vi "ExampleClient.vi"() -> ()   [LabVIEW 2017]
uses:
  Support/StreamClientState.ctl
  Controller/Support/StreamHeader.ctl
  jsonRPCwebservice/client/config.ctl
  Support/msg.ctl
  <userlib>/_SEH/Controls/CEH/CEH Actions.ctl
  <vilib>/NI/JSON Support for LabVIEW/JSON Data Classes/JSON String/JSON String.lvclass
  C:/Program Files (x86)/National Instruments/LabVIEW 2017/vi.lib/NI/JSON Support for LabVIEW/JSON Data Classes/JSON Datatype/JSON Null.lvclass
  Support/client_globals.vi
  jsonRPCwebservice/client/Request_int_JSON.vi
  <vilib>/NI/JSON Support for LabVIEW/JSON Data Classes/JSON Helper/To More Specific Type (Object).vi
  <vilib>/NI/JSON Support for LabVIEW/JSON Data Classes/JSON Object/Get Value (String).vi
  <vilib>/NI/JSON Support for LabVIEW/JSON Data Classes/JSON String/Read value (String).vi
  <vilib>/NI/JSON Support for LabVIEW/JSON Data Classes/JSON String/New JSON String.vi
  <vilib>/NI/JSON Support for LabVIEW/JSON Data Classes/JSON Helper/Parsing/Parse Value.vi
  <vilib>/NI/JSON Support for LabVIEW/JSON Data Classes/JSON Object/Get Value (Array).vi
  <vilib>/NI/JSON Support for LabVIEW/JSON Data Classes/JSON Array/Index Array XNode/index helper.vi
  <vilib>/NI/JSON Support for LabVIEW/JSON Data Classes/JSON Array/Index Array.vi
  <vilib>/NI/JSON Support for LabVIEW/JSON Data Classes/JSON Array/Index Array (JSON).vi
  <vilib>/NI/JSON Support for LabVIEW/JSON Data Classes/JSON Helper/To More Specific Type (Array).vi
  <vilib>/NI/JSON Support for LabVIEW/JSON Data Classes/JSON Array/Get Array Values as Strings.vi
  <vilib>/WebDAVClient/Simple Get File.vi
  <vilib>/NI/JSON Support for LabVIEW/JSON Data Classes/JSON Datatype/JSON Null.lvclass
  <vilib>/NI/JSON Support for LabVIEW/JSON Data Classes/JSON Array/Index Array XNode/Index JSON Array.xnode
  <vilib>/NI/JSON Support for LabVIEW/JSON Data Classes/JSON Array/JSON Array.lvclass
  jsonRPCwebservice/client/JSON_RPC_client.lvlib
  <vilib>/WebDAVClient/NI_WebDAV.lvlib
  <vilib>/NI/JSON Support for LabVIEW/JSON Data Classes/JSON Helper/JSON Helper.lvclass
  <vilib>/NI/JSON Support for LabVIEW/JSON Data Classes/JSON Object/JSON Object.lvclass
  <vilib>/NI/JSON Support for LabVIEW/JSON Data Classes/JSON Basic Type/JSON Literal.lvclass
panel:
  in  "Trace":string
  in  "Tab Control":enum32{"Commands", "Stream", "Files"}(tab)
  in  "ClearSafeState":bool
  in  "ToEcho":string
  in  "CheckConnection":bool
  in  "GoToSafeState":bool
  in  "GetResourceUsage":bool
  in  "echo":bool
  out "Current State":string
  out "logging":bool
  out "Waveforms":sgl[][](graph)
  in  "Stream":bool
  in  "StreamAndLog":bool
  in  "StopStreaming":bool
  in  "ForceTigger":bool
  in  "RefreshLogFiles":bool
  in  "Logs":i32(listbox)
  in  "Download":bool
  in  "Exit":bool
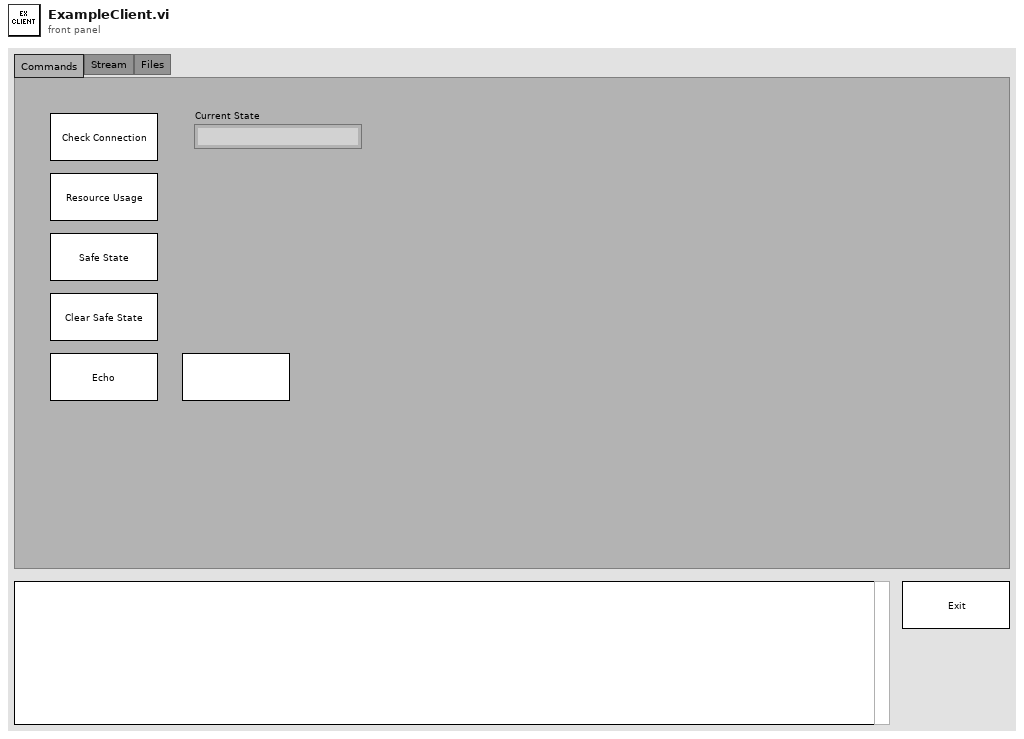
[diagram p1: front panel]
types:
  T1 = typedef "msg.ctl" = cluster{"cmd":string, "parameters":variant}
  T2 = typedef "JSON_RPC_client.lvlib/config.ctl" = cluster{"ip":string, "port":i32, "username":string, "password":string}
  T3 = typedef "StreamHeader.ctl" = cluster{"Channels":string[], "SampleRate":i32}
  T4 = typedef "StreamClientState.ctl" = enum16{"Initialize", "Idle", "ConnectAndOpen", "Connecting", "ReadHeader", "Streaming", "Disconnecting"}
  T5 = enum8{"Enabled", "Disabled", "Disabled and Grayed Out"}
  T6 = typedef "JSON_RPC_client.lvlib/reference.ctl" = cluster{"client handle":T7, "url":string}
  T7 = typedef "LabVIEWHTTPClient.lvlib/ClientHandle.ctl" = refnum<k1>
  T8 = enum16{"open", "open or create", "create or replace", "create", "open (read-only)"}
  T9 = typedef "SEH Notification Info.ctl" = cluster{"Priority":i32, "Occurrences":i32, "First Occurrence":timestamp}
  T10 = typedef "CEH Actions.ctl" = enum16{"Log", "Display Error Message", "Safe State", "Shutdown"}
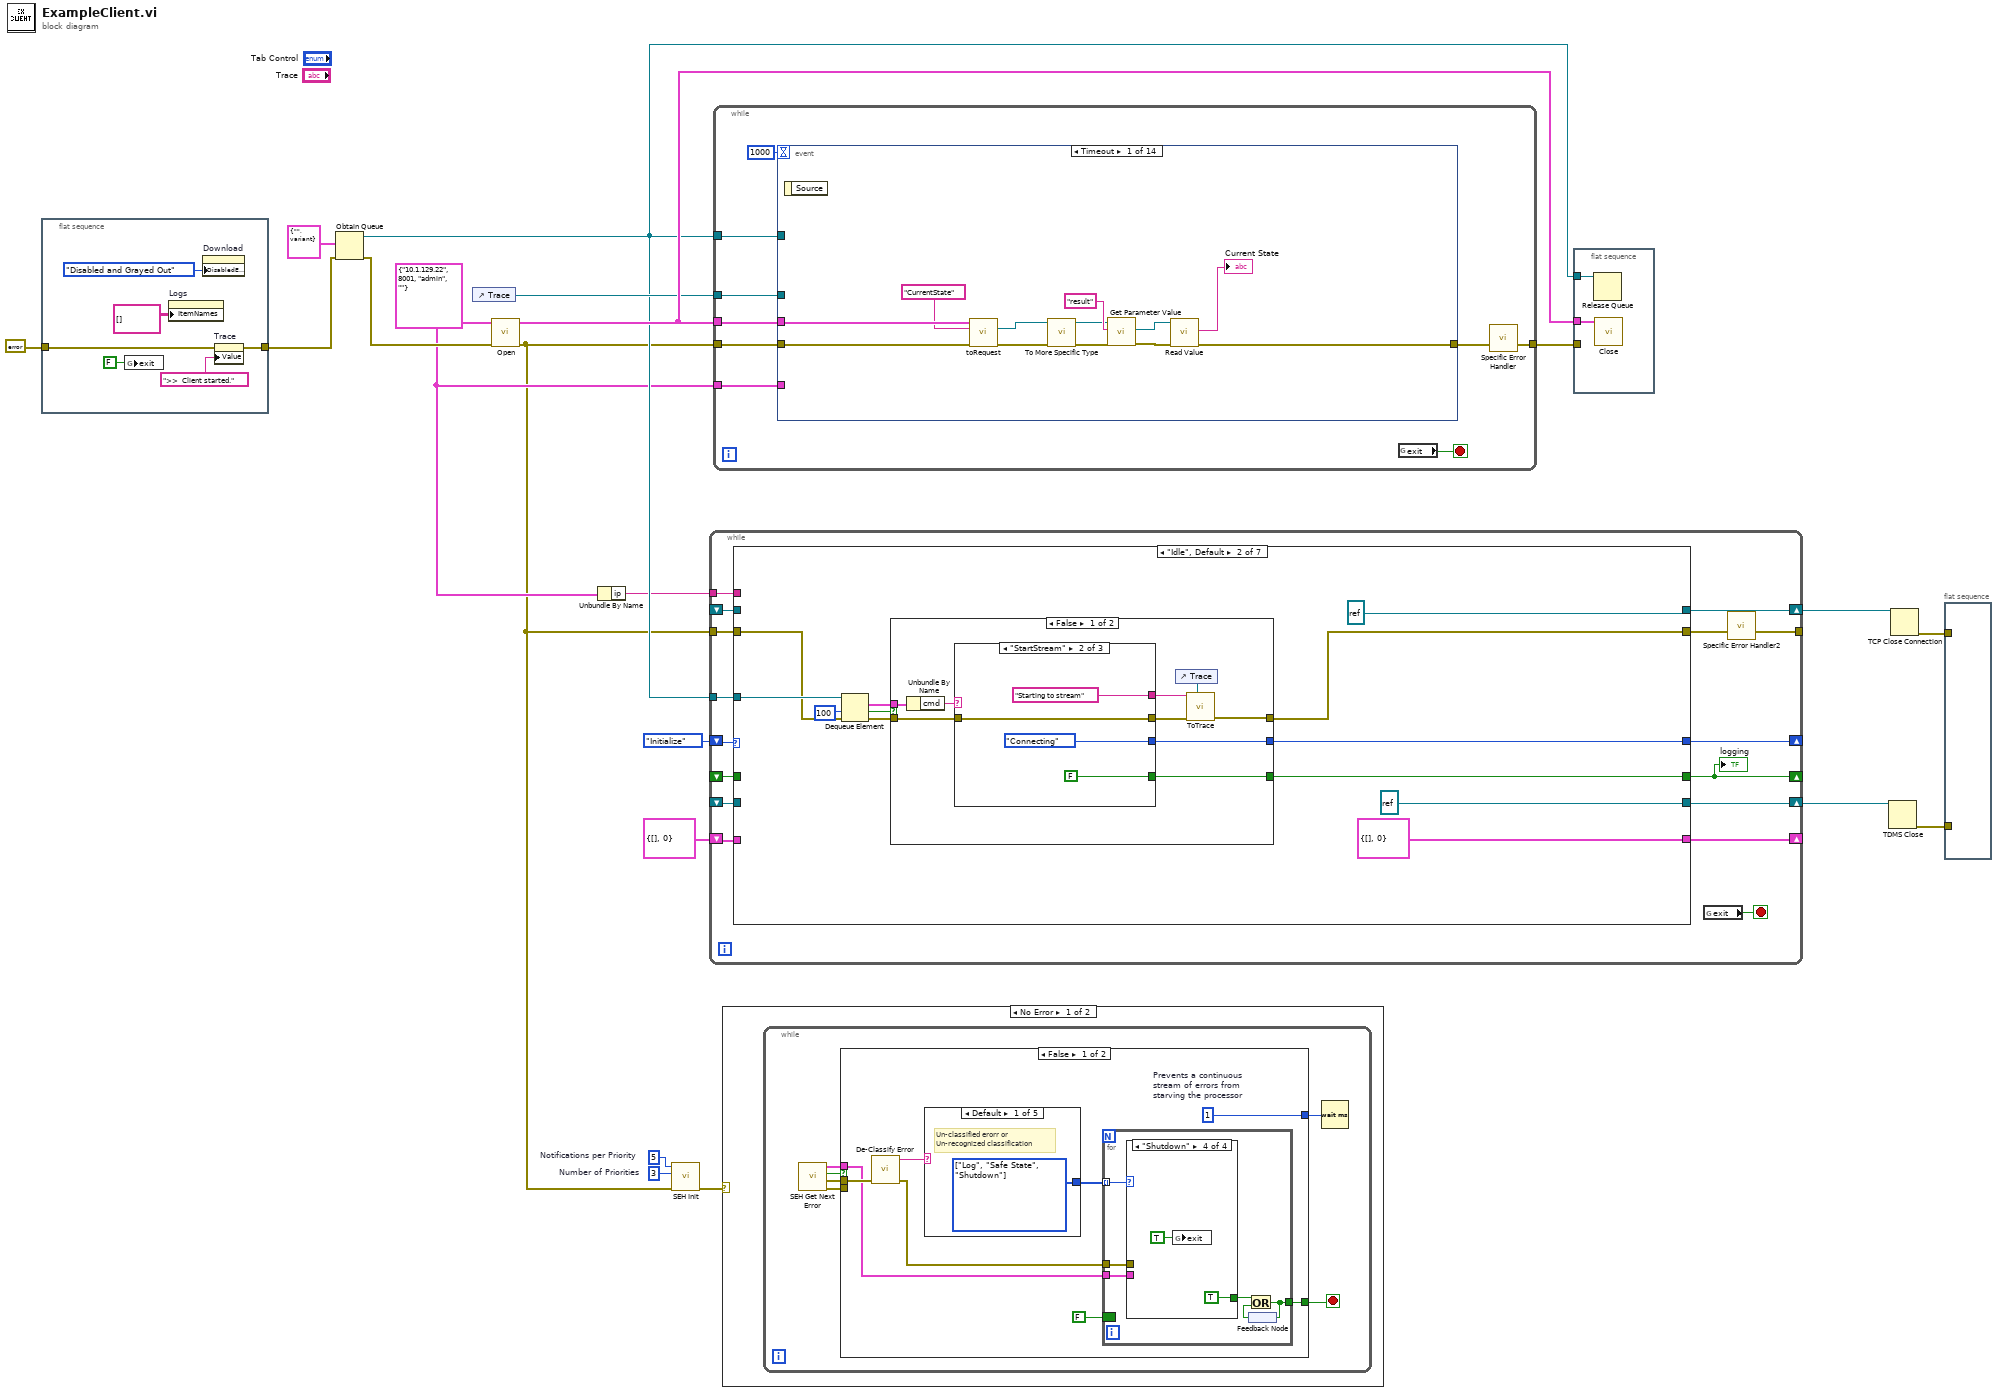
[diagram p0: block diagram]
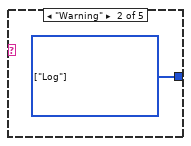
[diagram p2: hidden frame]
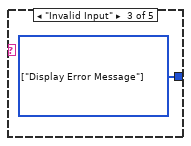
[diagram p3: hidden frame]
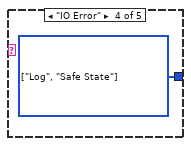
[diagram p4: hidden frame]
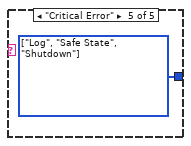
[diagram p5: hidden frame]
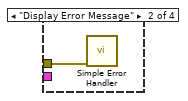
[diagram p7: hidden frame]
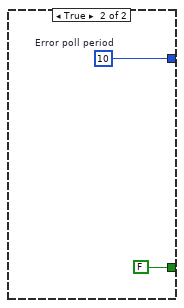
[diagram p9: hidden frame]
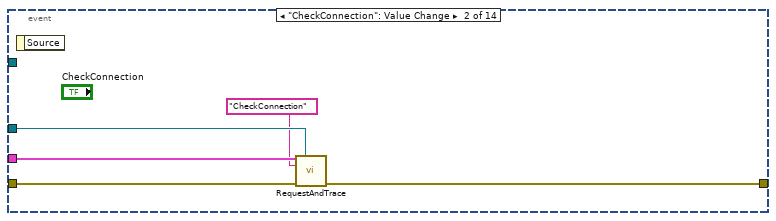
[diagram p11: hidden frame]
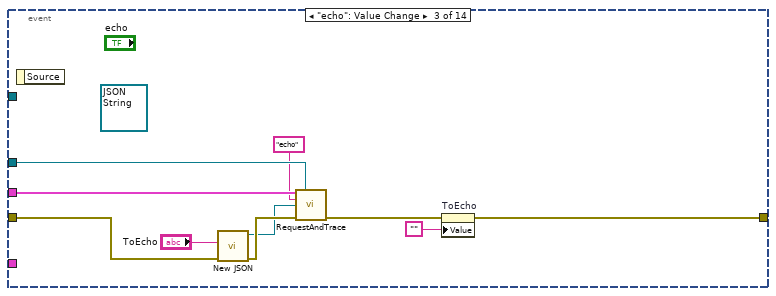
[diagram p12: hidden frame]
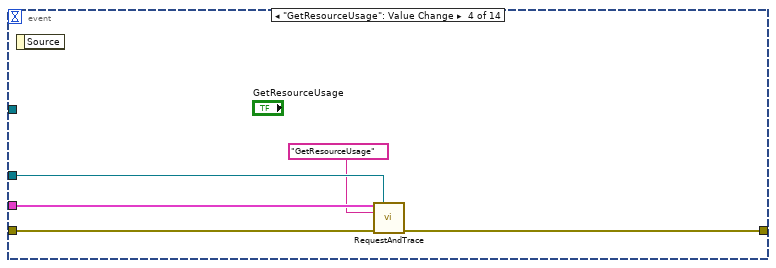
[diagram p13: hidden frame]
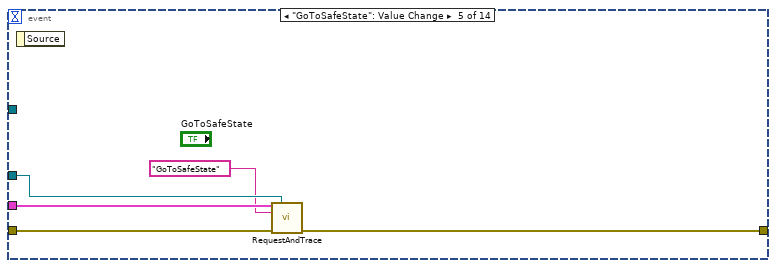
[diagram p14: hidden frame]
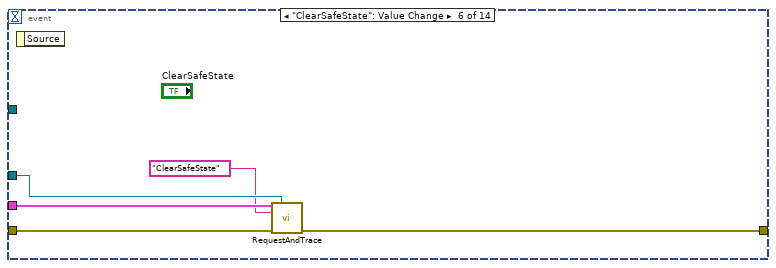
[diagram p15: hidden frame]
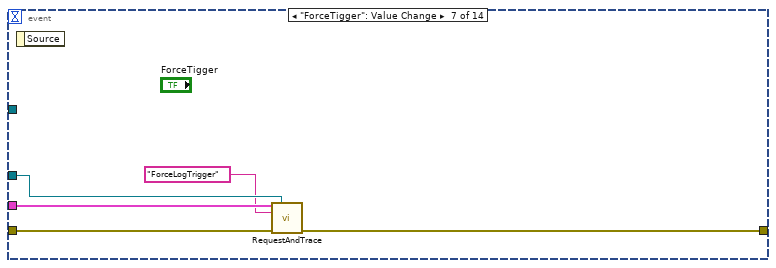
[diagram p16: hidden frame]
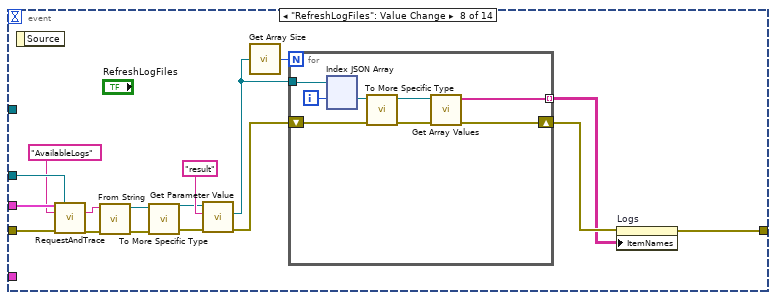
[diagram p17: hidden frame]
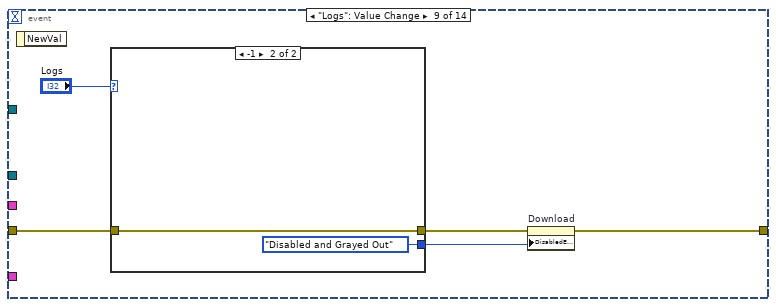
[diagram p18: hidden frame]
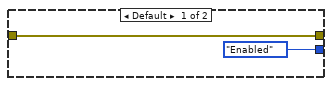
[diagram p19: hidden frame]
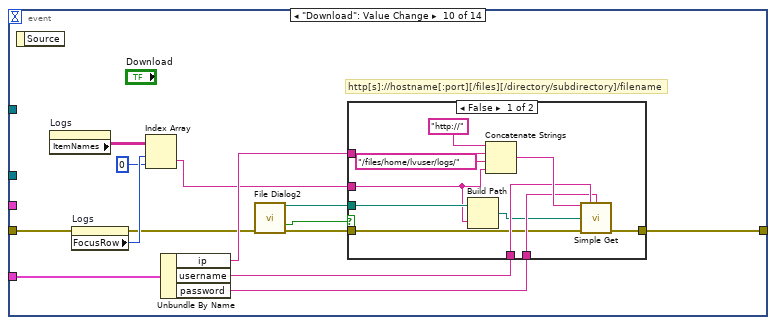
[diagram p20: hidden frame]
diagram:
  w8 = 3  # Number of Priorities
  w7 = 5  # Notifications per Priority
  w9 = T2 {"ip"="10.1.129.22", "port"=8001, "username"="admin", "password"=""} ("Connection")
  n1 = flat-sequence {
    tunnel: errorcluster {"status"=FALSE, "code"=0, "source"=""} ("error in (no error)") -> [w24]
    tunnel: [w23] -> w13
    frame #0 {
      n2 = global write "client_globals.vi" "exit"(FALSE ("exit")) -> ()
      n3 = property on="Logs" class="MCListbox (strict)"("ItemNames"=string[][] [] ("Item Names")) -> ()  [unwired: 2 in, 2 out]
      n4 = property on="Download" class="Bool"("DisabledEnum"=T5."Disabled and Grayed Out" ("Disabled")) -> ()  [unwired: 2 in, 2 out]
      n5 = property on="Trace" class="Str"(error in=w24, "Value"=">>  Client started." ("Trace")) -> (error out=w23:errorcluster)  [unwired: 1 in, 1 out]
    }
  }
  n6 = Obtain Queue(element data type=T1 {"cmd"="", "parameters"=variant} ("msg"), error in (no error)=w13) -> (queue out=w11:refnum<queue>, error out=w12:errorcluster)  [unwired: 3 in, 1 out]
  n7 = control-ref of="Trace"() -> (w15:refnum<vi>)
  n8 = call "Open.vi"("config"=w9, "error in (no error)"=w12) -> ("reference"=w18:T6, "error out"=w5:errorcluster)  [unwired: 12 in]
  n9 = Unbundle By Name(w9) -> ("ip"=w10:string)
  n10 = call <userlib>:"SEH Init.vi"("error in (no error)"=w5, "Number of Priorities"=w8, "Notifications per Priority"=w7) -> ("error out"=w6:errorcluster)  [unwired: 8 in]
  n11 = while {
    shift-right: [w41] -> _
    shift-left: StreamClientState."Initialize" ("StreamClientState") -> [w42]
    tunnel: w10 -> [w40]
    shift-right: [w38] -> w2
    shift-left: _ -> [w37]
    shift-right: [w36] -> _
    shift-left: T3 {"Channels"=[], "SampleRate"=0} ("StreamHeader") -> [w35]
    tunnel: w11 -> [w33]
    shift-right: [w27] -> _
    shift-left: _ -> [w32]
    shift-right: [w29] -> w1
    shift-left: _ -> [w28]
    tunnel: w5 -> [w39]
    tunnel: [w30] -> _
    stop <- w34 stop-if-true
    n12 = case shown="\"Idle\", Default" w42 {
      tunnel: [StreamClientState."Idle" ("StreamClientState") w66 w109 w139 w161 w199 StreamClientState."Idle" ("StreamClientState")] -> w41
      tunnel: w40 -> [_ _ w108 w144 _ _ _]
      tunnel: w39 -> [w45 w62 w104 w138 w173 w220 _]
      tunnel: [w53 w57 w95 w130 w162 w200 w229] -> w31
      tunnel: [refnum<k5> refnum ("connection ID") refnum<k5> refnum ("connection ID") w106 w141 w164 w210 refnum<k5> refnum ("connection ID")] -> w38
      tunnel: w37 -> [_ _ _ _ w172 w219 w242]
      tunnel: [T3 {"Channels"=[], "SampleRate"=0} ("StreamHeader") T3 {"Channels"=[], "SampleRate"=0} ("StreamHeader") _ _ w149 w206 _] -> w36
      tunnel: w35 -> [_ _ _ _ _ w206 _]
      tunnel: w33 -> [_ w63 _ _ _ w198 _]
      tunnel: [FALSE w56 w107 w137 w153 w203 FALSE] -> w27
      tunnel: w32 -> [_ _ w107 w137 w153 w203 _]
      tunnel: [refnum<k34> refnum ("tdms file out") refnum<k34> refnum ("tdms file out") w100 refnum<k34> refnum ("tdms file out") w151 w202 refnum<k34> refnum ("tdms file out")] -> w29
      tunnel: w28 -> [_ _ _ _ w152 w202 w236]
      frame "Initialize" {
        n13 = property on="StreamAndLog" class="Bool"(error in=w45, "DisabledEnum"=T5."Enabled" ("Disabled")) -> (error out=w47:errorcluster)  [unwired: 1 in, 1 out]
        n14 = property on="Stream" class="Bool"(error in=w47, "DisabledEnum"=T5."Enabled" ("Disabled")) -> (error out=w49:errorcluster)  [unwired: 1 in, 1 out]
        n15 = property on="StopStreaming" class="Bool"(error in=w49, "DisabledEnum"=T5."Disabled and Grayed Out" ("Disabled")) -> (error out=w53:errorcluster)  [unwired: 1 in, 1 out]
      }
      frame "Idle", Default {
        n16 = Dequeue Element(queue=w63, timeout in ms (-1)=100, error in (no error)=w62) -> (element=w59:T1, timed out?=w60:bool, error out=w58:errorcluster)  [unwired: 1 out]
        n17 = case shown="False" w60 {
          tunnel: [w75 StreamClientState."Idle" ("StreamClientState")] -> w66
          tunnel: w59 -> [w74 _]
          tunnel: w58 -> [w72 w91]
          tunnel: [w69 w91] -> w57
          tunnel: [w67 FALSE] -> w56
          frame False {
            n18 = Unbundle By Name(w74) -> ("cmd"=w73:string)
            n19 = case shown="\"StartStream\"" w73 {
              selector: w73 -> [w80 _ _]
              tunnel: [StreamClientState."Idle" ("StreamClientState") StreamClientState."Connecting" ("StreamClientState") StreamClientState."ConnectAndOpen" ("StreamClientState")] -> w75
              tunnel: w72 -> [w77 w83 w88]
              tunnel: [w78 "Starting to stream" "Starting to log streaming data"] -> w70
              tunnel: [w77 w83 w88] -> w68
              tunnel: [FALSE FALSE TRUE] -> w67
              frame Default {
                n20 = Concatenate Strings(w80, " command ignored" ("string")) -> (w78:string)
              }
              frame "StartStream" {
              }
              frame "StartStreamAndLog" {
              }
            }
            n21 = control-ref of="Trace"() -> (w71:refnum<vi>)
            n22 = call "ToTrace.vi"("ToTrace"=w70, "TraceRef"=w71, "error in (no error)"=w68) -> ("error out"=w69:errorcluster)  [unwired: 12 in]
          }
          frame True {
          }
        }
      }
      frame "ConnectAndOpen" {
        w94 = T5."Disabled and Grayed Out" ("Disabled")
        w99 = "*.tdms" ("pattern label")
        n23 = call "File Dialog"("prompt"="Select a new stream fie location", "error in"=w104, "pattern (all files)"=w99, "pattern label"=w99) -> ("selected path"=w101:path, "cancelled"=w102:bool, "error out"=w103:errorcluster)  [unwired: 8 in, 1 out]
        n24 = case shown="False" w102 {
          tunnel: [w119 errorcluster {"status"=FALSE, "code"=0, "source"=""} ("error IO")] -> w98
          tunnel: [w118 StreamClientState."Disconnecting" ("StreamClientState")] -> w109
          tunnel: w108 -> [w117 _]
          tunnel: [w116 refnum<k5> refnum ("connection ID")] -> w106
          tunnel: w103 -> [w115 _]
          tunnel: w101 -> [w113 _]
          tunnel: [w110 _] -> w100
          frame False {
            n25 = TDMS Open(5:FALSE ("create index file? (T)"), 8:w115, 10:T8."create or replace" ("operation (0:open)"), 11:w113) -> (0:w114:errorcluster, 3:w110:refnum<k34>)  [unwired: 3 in]
            n26 = TCP Open Connection(address=w117, remote port or service name=u16 55550, timeout ms (60000)=5000, error in (no error)=w114) -> (connection ID=w116:refnum<k5>, error out=w120:errorcluster)  [unwired: 1 in]
            n27 = case shown="Error" w120 {
              selector: w120 -> [w124 w126]
              tunnel: [w124 w126] -> w119
              tunnel: [StreamClientState."ReadHeader" ("StreamClientState") StreamClientState."Disconnecting" ("StreamClientState")] -> w118
              frame No Error {
              }
              frame Error {
              }
            }
          }
          frame True {
          }
        }
        n28 = property on="Stream" class="Bool"(error in=w98, "DisabledEnum"=w94) -> (error out=w97:errorcluster)  [unwired: 1 in, 1 out]
        n29 = property on="StreamAndLog" class="Bool"(error in=w97, "DisabledEnum"=w94) -> (error out=w96:errorcluster)  [unwired: 1 in, 1 out]
        n30 = property on="StopStreaming" class="Bool"(error in=w96, "DisabledEnum"=T5."Enabled" ("Disabled")) -> (error out=w95:errorcluster)  [unwired: 1 in, 1 out]
      }
      frame "Connecting" {
        w133 = T5."Disabled and Grayed Out" ("Disabled")
        n31 = TCP Open Connection(address=w144, remote port or service name=u16 55550, timeout ms (60000)=5000, error in (no error)=w138) -> (connection ID=w141:refnum<k5>, error out=w140:errorcluster)  [unwired: 1 in]
        n32 = case shown="No Error" w140 {
          selector: w140 -> [w146 w148]
          tunnel: [w146 w148] -> w134
          tunnel: [StreamClientState."ReadHeader" ("StreamClientState") StreamClientState."Disconnecting" ("StreamClientState")] -> w139
          frame No Error {
          }
          frame Error {
          }
        }
        n33 = property on="Stream" class="Bool"(error in=w134, "DisabledEnum"=w133) -> (error out=w135:errorcluster)  [unwired: 1 in, 1 out]
        n34 = property on="StreamAndLog" class="Bool"(error in=w135, "DisabledEnum"=w133) -> (error out=w132:errorcluster)  [unwired: 1 in, 1 out]
        n35 = property on="StopStreaming" class="Bool"(error in=w132, "DisabledEnum"=T5."Enabled" ("Disabled")) -> (error out=w130:errorcluster)  [unwired: 1 in, 1 out]
      }
      frame "ReadHeader" {
        w165 = 1000 ("timeout ms (25000)")
        n36 = TCP Read(connection ID=w172, bytes to read=4, error in (no error)=w173, 9:w165) -> (connection ID out=w167:refnum<k5>, data out=w170:string, error out=w168:errorcluster)  [unwired: 1 in]
        n37 = Type Cast(type=0, x=w170) -> (*(type *) &x=w166:i32)
        n38 = TCP Read(connection ID=w167, bytes to read=w166, error in (no error)=w168, 9:w165) -> (connection ID out=w164:refnum<k5>, data out=w160:string, error out=w163:errorcluster)  [unwired: 1 in]
        n39 = Unflatten From String(type=T3 {"Channels"=[], "SampleRate"=0} ("StreamHeader"), binary string=w160) -> (value=w149:T3)  [unwired: 3 in, 2 out]
        n40 = Unbundle By Name(w149) -> ("SampleRate"=w150:i32)
        n41 = Get Date/Time In Seconds() -> (seconds since 1Jan1904=w157:timestamp)
        n42 = Reciprocal(x=w150) -> (1/x=w158:dbl)
        n43 = To Variant(anything=w157) -> (Variant=w155:variant)
        n44 = To Variant(anything=w158) -> (Variant=w156:variant)
        n45 = Build Array(w156, w155) -> (w154:variant[])
        n46 = case shown="No Error" w163 {
          selector: w163 -> [w180 w191]
          tunnel: [w179 w191] -> w162
          tunnel: [StreamClientState."Streaming" ("StreamClientState") StreamClientState."Disconnecting" ("StreamClientState")] -> w161
          tunnel: w152 -> [w178 w190]
          tunnel: [w177 w190] -> w151
          tunnel: w154 -> [w176 _]
          tunnel: w153 -> [w175 _]
          tunnel: w149 -> [w174 _]
          frame No Error {
            n47 = Unbundle By Name(w174) -> ()  [unwired: 1 out]
            n48 = case shown="True" w175 {
              tunnel: w180 -> [w182 w189]
              tunnel: [w182 w188] -> w179
              tunnel: w178 -> [w183 w187]
              tunnel: [w183 w186] -> w177
              tunnel: w176 -> [_ w184]
              frame False {
              }
              frame True {
                n49 = TDMS Set Properties(5:w184, 7:string[] ["wf_increment", "wf_start_time"] ("property names"), 8:w189, 11:w187) -> (0:w188:errorcluster, 3:w186:refnum<k34>)  [unwired: 2 in, 2 out]
              }
            }
          }
          frame Error {
          }
        }
      }
      frame "Streaming" {
        w212 = 1000 ("timeout ms (25000)")
        n50 = Dequeue Element(queue=w198, timeout in ms (-1)=0) -> (element=w195:T1, error out=w196:errorcluster)  [unwired: 1 in, 2 out]
        n51 = Unbundle By Name(w195) -> ("cmd"=w194:string)
        n52 = case shown="\"\"" w194 {
          tunnel: w196 -> [_ _ _]
          tunnel: [StreamClientState."Streaming" ("StreamClientState") StreamClientState."Streaming" ("StreamClientState") StreamClientState."Disconnecting" ("StreamClientState")] -> w193
          frame Default {
          }
          frame "" {
          }
          frame "StopStream" {
          }
        }
        n53 = TCP Read(connection ID=w219, bytes to read=4, error in (no error)=w220, 9:w212) -> (connection ID out=w214:refnum<k5>, data out=w217:string, error out=w215:errorcluster)  [unwired: 1 in]
        n54 = Type Cast(type=0, x=w217) -> (*(type *) &x=w213:i32)
        n55 = TCP Read(connection ID=w214, bytes to read=w213, error in (no error)=w215, 9:w212) -> (connection ID out=w210:refnum<k5>, data out=w211:string, error out=w207:errorcluster)  [unwired: 1 in]
        n56 = Type Cast(type=sgl[] [], x=w211) -> (*(type *) &x=w208:sgl[])
        n57 = call "FormatWaveforms.vi"("WaveformArray"=w208, "logFileRef"=w202, "log"=w203, "StreamHeader"=w206, "error in (no error)"=w207) -> ("Waveforms"=w204:sgl[][], "UpdateWaveforms"=w205:bool, "error out"=w201:errorcluster)  [unwired: 8 in]
        n58 = case shown="True" w205 {
          tunnel: w204 -> [_ w228]
          frame False {
          }
          frame True {
            "Waveforms" <- w228
          }
        }
        n59 = case shown="Error" w201 {
          selector: w201 -> [w225 w227]
          tunnel: [w225 w227] -> w200
          tunnel: [w224 StreamClientState."Disconnecting" ("StreamClientState")] -> w199
          tunnel: w193 -> [w224 _]
          frame No Error {
          }
          frame Error {
          }
        }
      }
      frame "Disconnecting" {
        w231 = T5."Enabled" ("Disabled")
        n60 = TDMS Close(11:w236) -> (0:w238:errorcluster)  [unwired: 1 in, 1 out]
        n61 = TCP Close Connection(connection ID=w242) -> (error out=w239:errorcluster)  [unwired: 2 in, 1 out]
        n62 = flat-sequence {
          tunnel: w239 -> [_]
          tunnel: w238 -> [_]
          frame #0 {
          }
        }
        n63 = property on="Stream" class="Bool"(error in=errorcluster {"status"=FALSE, "code"=0, "source"=""} ("error IO"), "DisabledEnum"=w231) -> (error out=w234:errorcluster)  [unwired: 1 in, 1 out]
        n64 = property on="StreamAndLog" class="Bool"(error in=w234, "DisabledEnum"=w231) -> (error out=w233:errorcluster)  [unwired: 1 in, 1 out]
        n65 = property on="StopStreaming" class="Bool"(error in=w233, "DisabledEnum"=T5."Disabled and Grayed Out" ("Disabled")) -> (error out=w229:errorcluster)  [unwired: 1 in, 1 out]
      }
    }
    "logging" <- w27
    n66 = global read "client_globals.vi" "exit"() -> (w34:bool)
    n67 = call "Specific Error Handler2"("Error to Check"=w31) -> ("error out"=w30:errorcluster)  [unwired: 11 in, 3 out]
  }
  n68 = while {
    tunnel: w18 -> [w243]
    tunnel: w15 -> [w246]
    tunnel: w11 -> [w245]
    tunnel: w9 -> [w244]
    tunnel: w5 -> [w251]
    tunnel: [w247] -> w16
    stop <- w249 stop-if-true
    n69 = event shown="[0] Timeout" {
      selector: _ -> [_ _ _ _ _ _ _ _ _ _ _ _ _ _]
      dyn-events: _ -> [_ _ _ _ _ _ _ _ _ _ _ _ _ _]
      timeout: 1000 -> [_ _ _ _ _ _ _ _ _ _ _ _ _ _]
      tunnel: w243 -> [w262 w266 w278 w283 w288 w293 w298 w315 _ _ _ _ _ _]
      tunnel: w251 -> [w263 w268 w271 w282 w287 w292 w297 w314 w331 w351 w366 w372 w379 _]
      tunnel: [w252 w267 w275 w280 w285 w290 w295 w312 w332 w343 w365 w369 w375 errorcluster {"status"=TRUE, "code"=-1, "source"="User selected exit."} ("error out")] -> w248
      tunnel: w246 -> [_ w265 w277 w281 w286 w291 w296 w313 _ _ _ w368 w377 _]
      tunnel: w245 -> [_ _ _ _ _ _ _ _ _ _ w367 w373 w380 _]
      tunnel: w244 -> [_ _ _ _ _ _ _ _ _ w347 _ _ _ _]
      event Timeout {
        n70 = event-data() -> ()  [unwired: 1 in, 1 out]
        n71 = call-poly "toRequest.vi"("reference in"=w262, "method"="CurrentState" ("resulting string"), "error in (no error)"=w263) -> ("response"=w260:refnum<class "JSON Null.lvclass">, "error out"=w259:errorcluster)  [unwired: 10 in, 1 out]
        n72 = call-poly <vilib>:"To More Specific Type.vi"("error in (no error)"=w259, "JSON Datatype in"=w260) -> ("error out"=w256:errorcluster, "JSON Datatype out"=w257:refnum<class "JSON Object.lvclass">)  [unwired: 8 in]
        n73 = call-poly <vilib>:"Get Parameter Value.vi"("error in (no error)"=w256, "key"="result", "JSON Object in"=w257) -> ("error out"=w254:errorcluster, "value"=w255:refnum<class "JSON String.lvclass">)  [unwired: 7 in]
        n74 = call-poly <vilib>:"Read Value.vi"("error in (no error)"=w254, "JSON String in"=w255) -> ("error out"=w252:errorcluster, "value"=→"Current State":string)  [unwired: 8 in]
      }
      event "CheckConnection": Value Change {
        n75 = event-data() -> ()  [unwired: 1 in, 1 out]
        n76 = call "RequestAndTrace.vi"("JSONRef in"=w266, "TraceRef"=w265, "method"="CheckConnection" ("resulting string"), "error in (no error)"=w268) -> ("error out"=w267:errorcluster)  [unwired: 9 in, 2 out]
      }
      event "echo": Value Change {
        (unwired) refnum<class "JSON String.lvclass"> refnum ("JSON String out")
        n77 = event-data() -> ()  [unwired: 1 in, 1 out]
        n78 = call-poly <vilib>:"New JSON.vi"("error in (no error)"=w271, "value"="ToEcho") -> ("error out"=w270:errorcluster, "JSON String out"=w269:refnum<class "JSON String.lvclass">)  [unwired: 8 in]
        n79 = call "RequestAndTrace.vi"("JSONRef in"=w278, "TraceRef"=w277, "method"="echo" ("resulting string"), "params"=w269, "error in (no error)"=w270) -> ("error out"=w276:errorcluster)  [unwired: 8 in, 2 out]
        n80 = property on="ToEcho" class="Str"(error in=w276, "Value"="") -> (error out=w275:errorcluster)  [unwired: 1 in, 1 out]
      }
      event "GetResourceUsage": Value Change {
        n81 = event-data() -> ()  [unwired: 1 in, 1 out]
        n82 = call "RequestAndTrace.vi"("JSONRef in"=w283, "TraceRef"=w281, "method"="GetResourceUsage" ("resulting string"), "error in (no error)"=w282) -> ("error out"=w280:errorcluster)  [unwired: 9 in, 2 out]
      }
      event "GoToSafeState": Value Change {
        n83 = event-data() -> ()  [unwired: 1 in, 1 out]
        n84 = call "RequestAndTrace.vi"("JSONRef in"=w288, "TraceRef"=w286, "method"="GoToSafeState" ("resulting string"), "error in (no error)"=w287) -> ("error out"=w285:errorcluster)  [unwired: 9 in, 2 out]
      }
      event "ClearSafeState": Value Change {
        n85 = event-data() -> ()  [unwired: 1 in, 1 out]
        n86 = call "RequestAndTrace.vi"("JSONRef in"=w293, "TraceRef"=w291, "method"="ClearSafeState" ("resulting string"), "error in (no error)"=w292) -> ("error out"=w290:errorcluster)  [unwired: 9 in, 2 out]
      }
      event "ForceTigger": Value Change {
        n87 = event-data() -> ()  [unwired: 1 in, 1 out]
        n88 = call "RequestAndTrace.vi"("JSONRef in"=w298, "TraceRef"=w296, "method"="ForceLogTrigger" ("resulting string"), "error in (no error)"=w297) -> ("error out"=w295:errorcluster)  [unwired: 9 in, 2 out]
      }
      event "RefreshLogFiles": Value Change {
        n89 = event-data() -> ()  [unwired: 1 in, 1 out]
        n90 = call "RequestAndTrace.vi"("JSONRef in"=w315, "TraceRef"=w313, "method"="AvailableLogs" ("resulting string"), "error in (no error)"=w314) -> ("reponse"=w309:string, "error out"=w310:errorcluster)  [unwired: 9 in, 1 out]
        n91 = call <vilib>:"From String.vi"("error in (no error)"=w310, "JSON String"=w309) -> ("error out"=w302:errorcluster, "JSON out"=w301:refnum<class "JSON Null.lvclass">)  [unwired: 8 in]
        n92 = call-poly <vilib>:"To More Specific Type.vi"("error in (no error)"=w302, "JSON Datatype in"=w301) -> ("error out"=w299:errorcluster, "JSON Datatype out"=w300:refnum<class "JSON Object.lvclass">)  [unwired: 8 in]
        n93 = call-poly <vilib>:"Get Parameter Value.vi"("error in (no error)"=w299, "key"="result" ("Parameter Name"), "JSON Object in"=w300) -> ("error out"=w307:errorcluster, "value"=w304:refnum<class "JSON Array.lvclass">)  [unwired: 7 in]
        n94 = call <vilib>:"Get Array Size.vi"("JSON Array in"=w304) -> ("size(s)"=w305:i32)
        n95 = for {
          N: w305 -> [_]
          tunnel: w304 -> [w323]
          shift-right: [w317] -> w306
          shift-left: w307 -> [w320]
          tunnel: [w316] -> w303 mode=indexing
          i -> [w322]
          n96 = xnode "Index JSON Array"("index"=w322, "JSON Array In"=w323) -> ("element"=w321:refnum<class "JSON Null.lvclass">)  [unwired: 1 in, 1 out]
          n97 = call-poly <vilib>:"To More Specific Type.vi"("error in (no error)"=w320, "JSON Datatype in"=w321) -> ("error out"=w318:errorcluster, "JSON Datatype out"=w319:refnum<class "JSON Array.lvclass">)  [unwired: 8 in]
          n98 = call-poly <vilib>:"Get Array Values.vi"("error in (no error)"=w318, "JSON Array in"=w319) -> ("error out"=w317:errorcluster, "values"=w316:string[])  [unwired: 8 in]
        }
        n99 = property on="Logs" class="MCListbox (strict)"(error in=w306, "ItemNames"=w303) -> (error out=w312:errorcluster)  [unwired: 1 in, 1 out]
      }
      event "Logs": Value Change {
        n100 = event-data() -> ()  [unwired: 1 in, 1 out]
        n101 = case shown="-1" "Logs" {
          tunnel: w331 -> [w335 w336]
          tunnel: [w335 w336] -> w330
          tunnel: [T5."Enabled" ("Disabled") T5."Disabled and Grayed Out" ("Disabled")] -> w329
          frame Default {
          }
          frame -1 {
          }
        }
        n102 = property on="Download" class="Bool"(error in=w330, "DisabledEnum"=w329) -> (error out=w332:errorcluster)  [unwired: 1 in, 1 out]
      }
      event "Download": Value Change {
        # "http[s]://hostname[:port][/files][/directory/subdirectory]/filename"
        n103 = event-data() -> ()  [unwired: 1 in, 1 out]
        n104 = property on="Logs" class="MCListbox (strict)"() -> ("ItemNames"=w349:string[][])  [unwired: 2 in, 2 out]
        n105 = property on="Logs" class="MCListbox (strict)"(error in=w351) -> (error out=w342:errorcluster, "FocusRow"=w350:i32)  [unwired: 1 in, 1 out]
        n106 = Index Array(array=w349, index (row)=w350, index (col)=0 ("index")) -> (element=w340:string)
        n107 = Unbundle By Name(w347) -> ("ip"=w346:string, "username"=w345:string, "password"=w344:string)
        n108 = call "File Dialog2"("error in"=w342) -> ("selected path"=w341:path, "cancelled"=w338:bool, "error out"=w339:errorcluster)  [unwired: 11 in, 1 out]
        n109 = case shown="False" w338 {
          tunnel: w346 -> [w361 _]
          tunnel: w345 -> [w358 _]
          tunnel: w344 -> [w357 _]
          tunnel: [w356 w363] -> w343
          tunnel: w341 -> [w355 _]
          tunnel: w340 -> [w354 _]
          tunnel: w339 -> [w352 w363]
          frame False {
            n110 = Build Path(base path=w355, name or relative path=w354) -> (appended path=w353:path)
            n111 = Concatenate Strings("http://" ("string"), w361, "/files/home/lvuser/logs/" ("string"), w354) -> (w359:string)
            n112 = call-poly <vilib>:"Simple Get.vi"("remote file uri"=w359, "username"=w358, "password"=w357, "local file path"=w353, "error in (no error)"=w352) -> ("error out"=w356:errorcluster)  [unwired: 9 in, 1 out]
          }
          frame True {
          }
        }
      }
      event "Stream": Value Change {
        n113 = event-data() -> ()  [unwired: 1 in, 1 out]
        n114 = Enqueue Element(queue=w367, element=T1 {"cmd"="StartStream", "parameters"=variant}, error in (no error)=w366) -> (error out=w365:errorcluster)  [unwired: 1 in, 2 out]
      }
      event "StreamAndLog": Value Change {
        n115 = event-data() -> ()  [unwired: 1 in, 1 out]
        n116 = Enqueue Element(queue=w373, element=T1 {"cmd"="StartStreamAndLog", "parameters"=variant}, error in (no error)=w372) -> (error out=w370:errorcluster)  [unwired: 1 in, 2 out]
        n117 = call "ToTrace.vi"("ToTrace"="Stream and log started.", "TraceRef"=w368, "error in (no error)"=w370) -> ("error out"=w369:errorcluster)  [unwired: 12 in]
      }
      event "StopStreaming": Value Change {
        n118 = event-data() -> ()  [unwired: 1 in, 1 out]
        n119 = Enqueue Element(queue=w380, element=T1 {"cmd"="StopStream", "parameters"=variant}, error in (no error)=w379) -> (error out=w378:errorcluster)  [unwired: 1 in, 2 out]
        n120 = call "ToTrace.vi"("ToTrace"="Streaming stopped.", "TraceRef"=w377, "error in (no error)"=w378) -> ("error out"=w375:errorcluster)  [unwired: 12 in]
      }
      event "Exit": Value Change {
        n121 = event-data() -> ()  [unwired: 1 in, 1 out]
      }
    }
    n122 = global read "client_globals.vi" "exit"() -> (w249:bool)
    n123 = call "Specific Error Handler"("Error to Check"=w248) -> ("error out"=w247:errorcluster)  [unwired: 11 in, 3 out]
  }
  n124 = case shown="No Error" w6 {
    frame No Error {
      n125 = while {
        stop <- w387 stop-if-true
        n126 = call <userlib>:"SEH Get Next Error.vi"() -> ("Transmission Error"=w383:errorcluster, "Transmitted Error"=w386:errorcluster, "Empty?"=w385:bool, "Notification Info"=w384:T9)  [unwired: 8 in]
        n127 = case shown="False" w385 {
          tunnel: [w396 w412] -> w388
          tunnel: w386 -> [w395 _]
          tunnel: w384 -> [w391 _]
          tunnel: [w390 FALSE] -> w387
          tunnel: w383 -> [_ _]
          frame False {
            w396 = u32 1  # Prevents a continuous stream of errors from starving the processor
            n128 = call <userlib>:"De-Classify Error.vi"("Classified Error"=w395) -> ("De-Classified Error"=w393:errorcluster, "Error Classification"=w394:string)  [unwired: 8 in, 1 out]
            n129 = case shown="Default" w394 {
              tunnel: [w397 w398 w399 w400 w401] -> w392
              frame Default {
                w397 = T10[] [enum."Log", enum."Safe State", enum."Shutdown"] items=["Log", "Display Error Message", "Safe State", "Shutdown"]
                # "Un-classified erorr or\nUn-recognized classification"
              }
              frame "Warning" {
                w398 = T10[] [enum."Log"] items=["Log", "Display Error Message", "Safe State", "Shutdown"]
              }
              frame "Invalid Input" {
                w399 = T10[] [enum."Display Error Message"] items=["Log", "Display Error Message", "Safe State", "Shutdown"]
              }
              frame "IO Error" {
                w400 = T10[] [enum."Log", enum."Safe State"] items=["Log", "Display Error Message", "Safe State", "Shutdown"]
              }
              frame "Critical Error" {
                w401 = T10[] [enum."Log", enum."Safe State", enum."Shutdown"] items=["Log", "Display Error Message", "Safe State", "Shutdown"]
              }
            }
            n130 = for {
              tunnel: w393 -> [w406]
              tunnel: w392 -> [w407] mode=indexing
              tunnel: w391 -> [w405]
              border: FALSE -> [_]
              tunnel: [w402] -> w390
              n131 = case shown="\"Shutdown\"" w407 {
                tunnel: w406 -> [_ w408 _ _]
                tunnel: w405 -> [_ _ _ _]
                tunnel: [_ _ _ TRUE] -> w404
                frame "Log", Default {
                  # "Implement log \nhere"
                }
                frame "Display Error Message" {
                  n132 = call <vilib>:"Simple Error Handler.vi"("error in (no error)"=w408) -> ()  [unwired: 4 in, 5 out]
                }
                frame "Safe State" {
                  # "Implement safe\nstate here"
                }
                frame "Shutdown" {
                  n133 = global write "client_globals.vi" "exit"(TRUE ("exit")) -> ()
                }
              }
              n134 = feedback #1() -> (w403:bool)
              n135 = Or(x=w404, y=w403) -> (x .or. y?=w402:bool)
              n136 = feedback-in #1(w402) -> ()
            }
          }
          frame True {
            w412 = u32 10  # Error poll period
          }
        }
        n137 = Wait (ms)(milliseconds to wait=w388) -> ()  [unwired: 1 out]
      }
    }
    frame Error {
      # "Error notification cannot initialize\n(log this)"
    }
  }
  n138 = flat-sequence {
    tunnel: w18 -> [w414]
    tunnel: w16 -> [_]
    tunnel: w11 -> [w413]
    frame #0 {
      n139 = Release Queue(queue=w413) -> ()  [unwired: 2 in, 3 out]
      n140 = call "Close.vi"("reference in"=w414) -> ()  [unwired: 14 in, 1 out]
    }
  }
  n141 = TDMS Close(11:w1) -> (0:w3:errorcluster)  [unwired: 1 in, 1 out]
  n142 = TCP Close Connection(connection ID=w2) -> (error out=w4:errorcluster)  [unwired: 2 in, 1 out]
  n143 = flat-sequence {
    tunnel: w4 -> [_]
    tunnel: w3 -> [_]
    frame #0 {
    }
  }
